vi "Video(new).vi"(8 "error in (no error)":errorcluster, 11 "AR Drone Resource":T1={"UDP Control Connection"=refnum, "UDP NavData Connection"=refnum, "UDP Video Connection (Drone 1.0)"=refnum, "TCP Video Connection (Drone 2.0)"=refnum, "TCP Control Port Connection"=refnum, "Drone IP address"="192.168.1.1", "Drone Command Port"=5555, "Drone NavData Port"=5555, "Drone Vid Stream Port"=56828, "Drone TCP Control Port"=5559, "Home IP address"="192.168.1.2", "Home Command Port"=56829, "Home NavData Port"=56830, "Home Vid Stream Port"=0, "Drone Version"=0, "Drone Index"=0, "Command Sequence"=1}) -> (0 "error out":errorcluster, 1 "Video Data Out (2.0)":u8[](array[numeric]), 2 "AR Drone Resource Out":T1={"UDP Control Connection"=refnum, "UDP NavData Connection"=refnum, "UDP Video Connection (Drone 1.0)"=refnum, "TCP Video Connection (Drone 2.0)"=refnum, "TCP Control Port Connection"=refnum, "Drone IP address"="192.168.1.1", "Drone Command Port"=5555, "Drone NavData Port"=5555, "Drone Vid Stream Port"=56828, "Drone TCP Control Port"=5559, "Home IP address"="192.168.1.2", "Home Command Port"=56829, "Home NavData Port"=56830, "Home Vid Stream Port"=0, "Drone Version"=0, "Drone Index"=0, "Command Sequence"=1}, 3 "Video Stream":picture)   [LabVIEW 2014]
doc: "Very simple example showing how to use the base VIs to control the AR Drone and receive and display video data."
uses:
  <vilib>/picture/picture.llb/Draw True-Color Pixmap.vi
  Drone Project/AR Drone Toolkit (BETA)/Decode Video/2.0/Decode20Video.dll
  <vilib>/LVH/AR Drone Toolkit/Type Defs/AR Drone Resource.ctl
  <vilib>/LVH/AR Drone Toolkit/AR Drone.lvlib
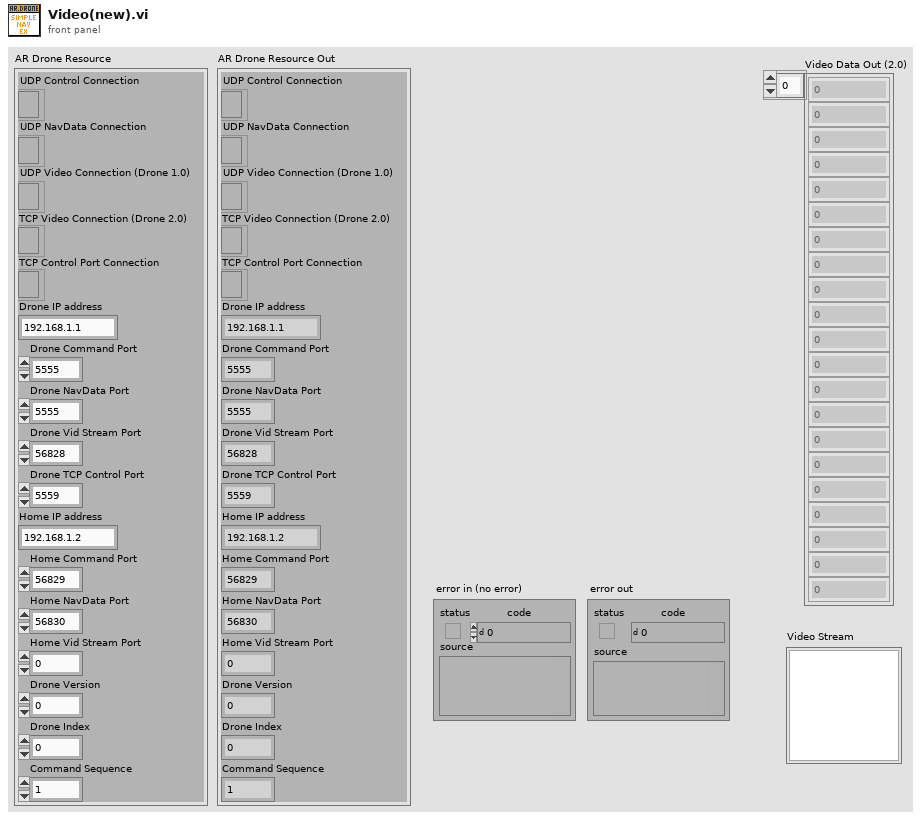
[diagram p1: front panel]
types:
  T1 = typedef "AR Drone.lvlib/AR Drone Resource.ctl" = cluster{"UDP Control Connection":refnum<k16>, "UDP NavData Connection":refnum<k16>, "UDP Video Connection (Drone 1.0)":refnum<k16>, "TCP Video Connection (Drone 2.0)":refnum<k5>, "TCP Control Port Connection":refnum<k5>, "Drone IP address":string, "Drone Command Port":u16, "Drone NavData Port":u16, "Drone Vid Stream Port":u16, "Drone TCP Control Port":u16, "Home IP address":string, "Home Command Port":u16, "Home NavData Port":u16, "Home Vid Stream Port":u16, "Drone Version":i32, "Drone Index":i32, "Command Sequence":i32}
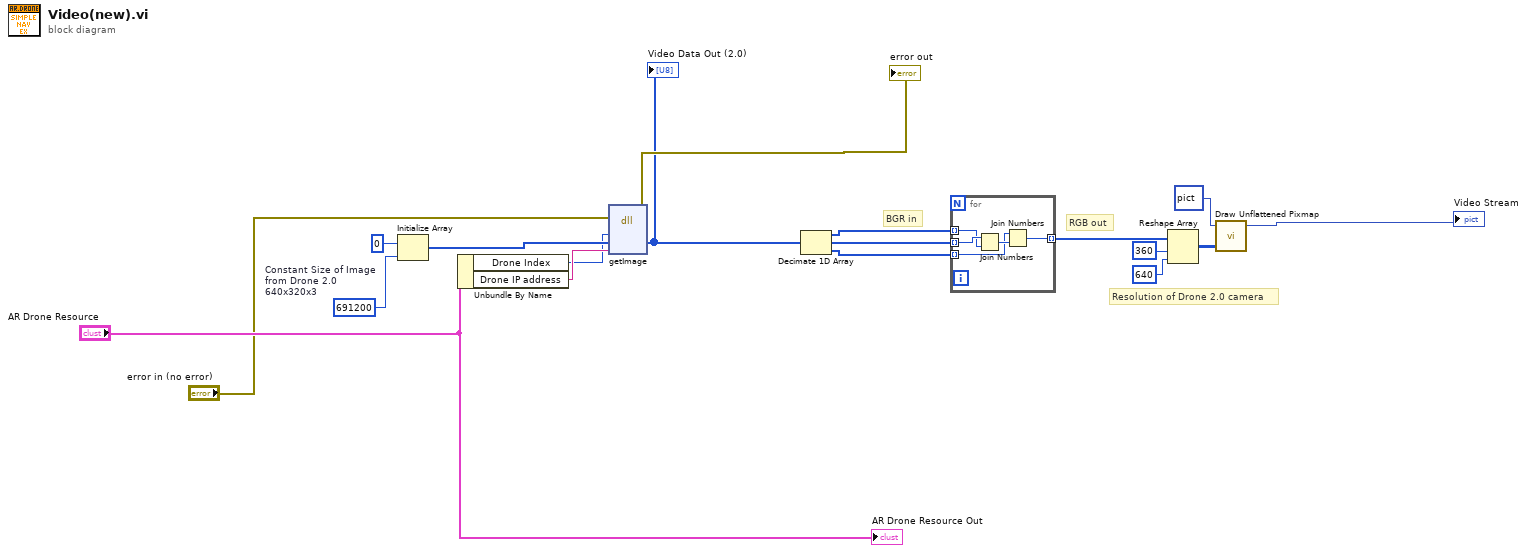
[diagram p0: block diagram]
diagram:
  w15 = 691200  # Constant Size of Image from Drone 2.0 640x320x3
  # "Resolution of Drone 2.0 camera"
  # "RGB out"
  # "BGR in"
  n1 = Initialize Array(u8 0 ("dimension size"), w15) -> (w13:u8[])
  n2 = Unbundle By Name("AR Drone Resource") -> ("Drone Index"=w11:i32, "Drone IP address"=w12:string)
  n3 = dll-call lib="E:/Dropbox/UTCN/Summer 2015/Drone Project/AR Drone Toolkit (BETA)/Decode Video/2.0/Decode20Video.dll" fn="getImage"(error in="error in (no error)", "Index"=w11, "ImgData"=w13, "IP Address"=w12) -> (error out=→"error out":errorcluster, "ImgData"=w2:u8[])  [unwired: 5 in, 1 out]
  "Video Data Out (2.0)" <- w2
  n4 = Decimate 1D Array(w2) -> (w5:u8[], w4:u8[], w3:u8[])
  n5 = for {
    tunnel: [w22] -> w10 mode=indexing
    tunnel: w5 -> [w20] mode=indexing
    tunnel: w4 -> [w21] mode=indexing
    tunnel: w3 -> [w19] mode=indexing
    n6 = Join Numbers(hi=w21, lo=w20) -> ((hi.lo)=w23:u16)
    n7 = Join Numbers(hi=w19, lo=w23) -> ((hi.lo)=w22:u32)
  }
  n8 = Reshape Array(w10, 360 ("dimension size"), 640 ("dimension size")) -> (w9:u32[][])
  n9 = call-poly <vilib>:"Draw Unflattened Pixmap.vi"("picture"=picture data[5B], "data (RGB format)"=w9) -> ("new picture"=→"Video Stream":picture)  [unwired: 7 in]
  "AR Drone Resource Out" <- "AR Drone Resource"
